vi "put_cushion.vi"(8 "error in (no error)":errorcluster, 11 "ChairWithTableAttached.lvclass":refnum<class "ChairWithTableAttached.lvclass">) -> (0 "error out":errorcluster, 1 "result":string, 3 "ChairWithTableAttached.lvclass":refnum<class "ChairWithTableAttached.lvclass">)   [LabVIEW 2021, in "ChairWithTableAttached.lvclass"]
uses:
  ChairWithTableAttached.lvclass
  ChairWithTableAttached.lvclass/ChairWithTableAttached.ctl
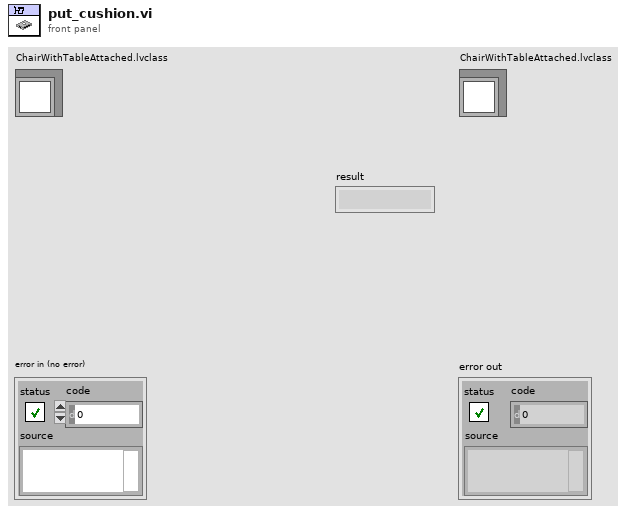
[diagram p1: front panel]
types:
  T1 = typedef "IChair.lvclass/CushionModel.ctl" = u16
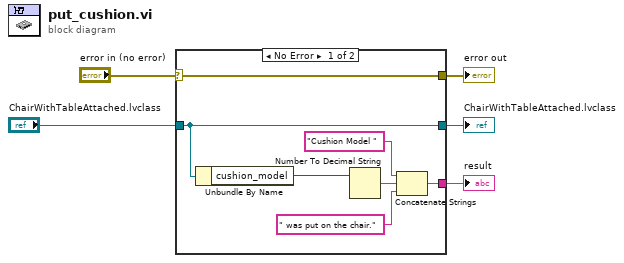
[diagram p0: block diagram]
diagram:
  n1 = case shown="No Error" "error in (no error)" {
    selector: "error in (no error)" -> [w12 w14]
    tunnel: [w12 w14] -> w4
    tunnel: [w11 w13] -> w2
    tunnel: "ChairWithTableAttached.lvclass" -> [w11 w13]
    tunnel: [w6 _] -> w1
    frame No Error {
      n2 = Unbundle By Name(w11) -> ("cushion_model"=w7:T1)
      n3 = Number To Decimal String(number=w7) -> (decimal integer string=w8:string)  [unwired: 1 in]
      n4 = Concatenate Strings("Cushion Model ", w8, " was put on the chair.") -> (w6:string)
    }
    frame Error {
    }
  }
  "error out" <- w4
  "ChairWithTableAttached.lvclass" <- w2
  "result" <- w1
